vi "elementAttributeAdd.vi"(0 "DOM document in":refnum<k20>, 5 "elementName":string, 7 "property":string[](array[string]), 9 "value":string[](array[string]), 11 "错误输入（无错误）":errorcluster) -> (4 "DOM document out":refnum<k20>, 6 "element":refnum<k20>, 15 "错误输出":errorcluster)   [LabVIEW 2011]
uses:
  C:/Program Files (x86)/National Instruments/LabVIEW 2011/resource/objmgr/DOMUserDefRef.rc
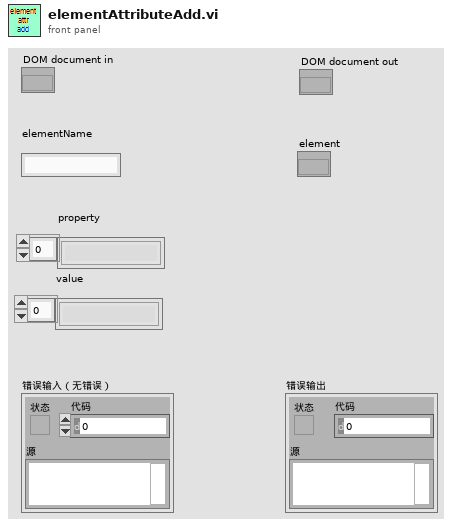
[diagram p1: front panel]
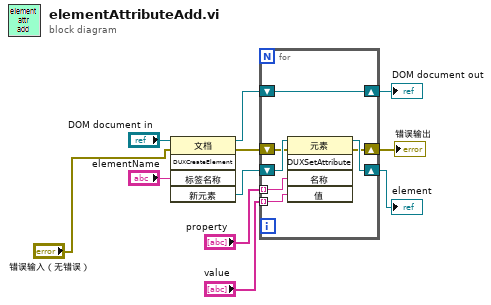
[diagram p0: block diagram]
diagram:
  n1 = invoke class="文档" method="DUXCreateElement"(reference="DOM document in", error in="错误输入（无错误）", "标签名称"="elementName") -> (reference out=w3:refnum<k20>, error out=w7:errorcluster, "新元素"=w10:refnum<k20>)  [unwired: 2 in, 2 out]
  n2 = for {
    shift-right: [w17] -> w5
    shift-left: w10 -> [w18]
    tunnel: "property" -> [w16] mode=indexing
    tunnel: "value" -> [w15] mode=indexing
    shift-right: [w13] -> w6
    shift-left: w7 -> [w14]
    shift-right: [w12] -> w2
    shift-left: w3 -> [w12]
    n3 = invoke class="元素" method="DUXSetAttribute"(reference=w18, error in=w14, "名称"=w16, "值"=w15) -> (reference out=w17:refnum<k20>, error out=w13:errorcluster)  [unwired: 1 in, 3 out]
  }
  "错误输出" <- w6
  "element" <- w5
  "DOM document out" <- w2
